vi "Tektronix_Read_Measurement (2 Channels).vi"(6 "Measurement Type (0: Phase)":i32(ring) items=["Phase", "Delay", "DelayRR", "DelayRF", "DelayFR", "DelayFF"], 7 "Oscilloscope-Change":bool=TRUE, 8 "error in (no error)":errorcluster, 9 "Channel 2 (2: Channel 2)":i32(ring)=2 items=["Channel 1"=1, "Channel 2"=2, "Channel 3"=3, "Channel 4"=4], 10 "Channel 1 (1: Channel 1)":i32(ring)=1 items=["Channel 1"=1, "Channel 2"=2, "Channel 3"=3, "Channel 4"=4], 11 "TestIndex":i32) -> (0 "error out":errorcluster, 1 "Units":string, 2 "Measurement":dbl, 3 "VISA resource name out":refnum<visa-resource-name>)   [LabVIEW 2015]
doc: "This VI displays the results of the selected 2 channels measurement."
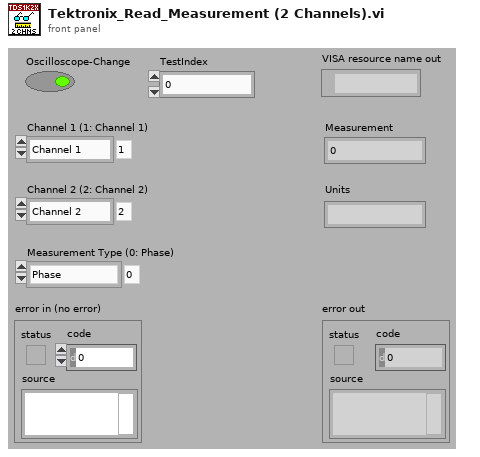
[diagram p1: front panel]
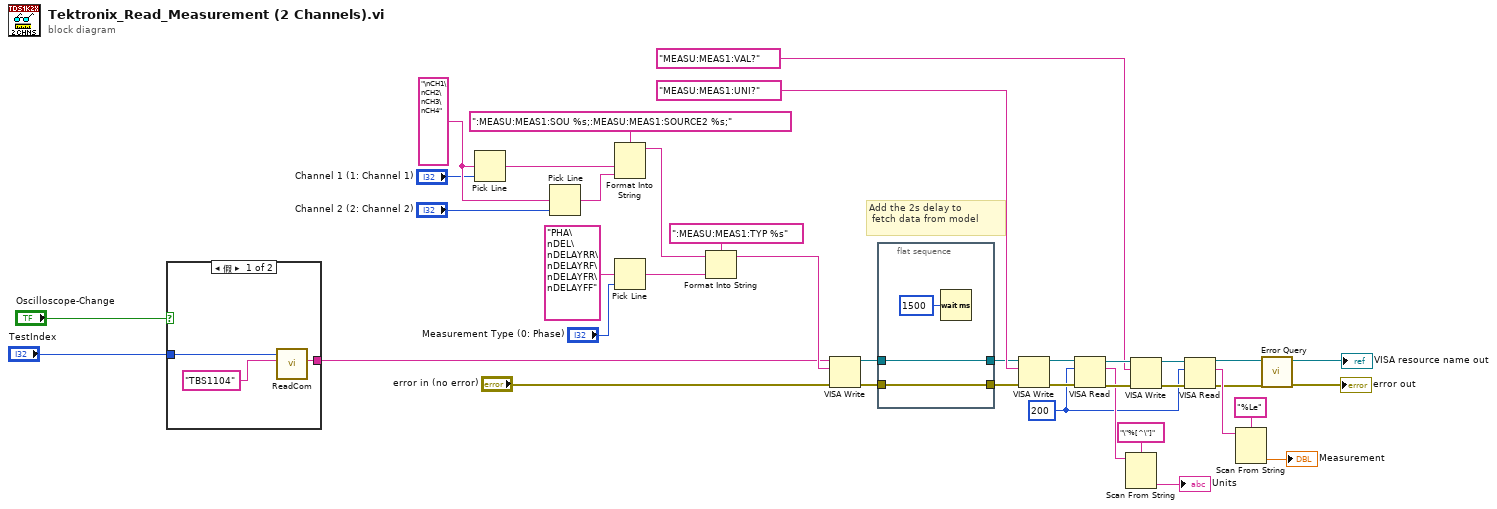
[diagram p0: block diagram]
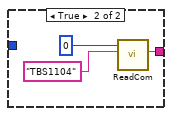
[diagram p2: hidden frame]
diagram:
  w4 = u32 200 ("byte count")
  w23 = "\nCH1\nCH2\nCH3\nCH4"
  # "Add the 2s delay to\n fetch data from model"
  n1 = case shown="假" "Oscilloscope-Change" {
    tunnel: "TestIndex" -> [w40 _]
    tunnel: [w41 w43] -> w1
    frame False {
      n2 = call "ReadCom.vi"("仪器名称"="TBS1104", "MyIndex"=w40) -> ("COM"=w41:string)  [unwired: 7 in, 2 out]
    }
    frame True {
      n3 = call "ReadCom.vi"("仪器名称"="TBS1104", "MyIndex"=u8 0) -> ("COM"=w43:string)  [unwired: 7 in, 2 out]
    }
  }
  n4 = Pick Line(multi-line string=w23, line index="Channel 1 (1: Channel 1)") -> (output string=w21:string)  [unwired: 1 out]
  n5 = Pick Line(multi-line string=w23, line index="Channel 2 (2: Channel 2)") -> (output string=w22:string)  [unwired: 1 out]
  n6 = Format Into String(format string=":MEASU:MEAS1:SOU %s;:MEASU:MEAS1:SOURCE2 %s;", w21, w22) -> (resulting string=w7:string)  [unwired: 2 in, 1 out]
  n7 = Pick Line(multi-line string="PHA\nDEL\nDELAYRR\nDELAYRF\nDELAYFR\nDELAYFF", line index="Measurement Type (0: Phase)") -> (output string=w9:string)  [unwired: 1 out]
  n8 = Format Into String(format string=":MEASU:MEAS1:TYP %s", initial string=w7, w9) -> (resulting string=w6:string)  [unwired: 1 in, 1 out]
  n9 = VISA Write(VISA resource name=w1, write buffer=w6, error in (no error)="error in (no error)") -> (VISA resource name out=w14:refnum<visa-resource-name>, error out=w13:errorcluster)  [unwired: 1 out]
  n10 = flat-sequence {
    tunnel: w14 -> [w47]
    tunnel: w13 -> [w48]
    tunnel: [w48] -> w12
    tunnel: [w47] -> w11
    frame #0 {
      n11 = Wait (ms)(milliseconds to wait=u32 1500) -> ()  [unwired: 1 out]
    }
  }
  n12 = VISA Write(VISA resource name=w11, write buffer="MEASU:MEAS1:UNI?", error in (no error)=w12) -> (VISA resource name out=w39:refnum<visa-resource-name>, error out=w38:errorcluster)  [unwired: 1 out]
  n13 = VISA Read(VISA resource name=w39, byte count=w4, error in (no error)=w38) -> (VISA resource name out=w34:refnum<visa-resource-name>, read buffer=w29:string, error out=w33:errorcluster)  [unwired: 1 out]
  n14 = Scan From String(format string="\"%[^\"]", input string=w29) -> (output 1=→"Units":string)  [unwired: 2 in, 4 out]
  n15 = VISA Write(VISA resource name=w34, write buffer="MEASU:MEAS1:VAL?", error in (no error)=w33) -> (VISA resource name out=w36:refnum<visa-resource-name>, error out=w35:errorcluster)  [unwired: 1 out]
  n16 = VISA Read(VISA resource name=w36, byte count=w4, error in (no error)=w35) -> (VISA resource name out=w18:refnum<visa-resource-name>, read buffer=w31:string, error out=w17:errorcluster)  [unwired: 1 out]
  n17 = Scan From String(format string="%Le", input string=w31) -> (output 1=→"Measurement":dbl)  [unwired: 2 in, 4 out]
  n18 = call "Error Query.vi"("error in (no error)"=w17, "VISA resource name"=w18) -> ("error out"=→"error out":errorcluster, "VISA resource name out"=→"VISA resource name out":refnum<visa-resource-name>)  [unwired: 8 out]
